vi "set initial operation mode.vi"(8 "error in (no error)":errorcluster, 11 "CCDCamera in":refnum<class "iKon-L.lvclass">) -> (0 "error out":errorcluster, 3 "CCDCamera out":refnum<class "iKon-L.lvclass">)   [LabVIEW 2018, in "iKon-L.lvclass"]
doc: "Write the current operation mode to the camera"
uses:
  iKon-L.lvclass
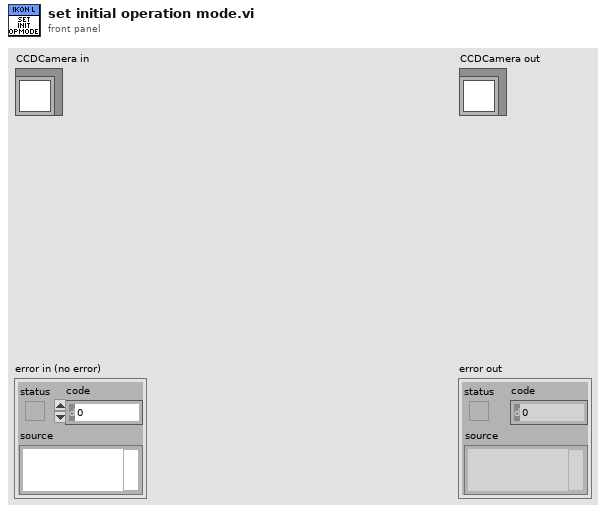
[diagram p1: front panel]
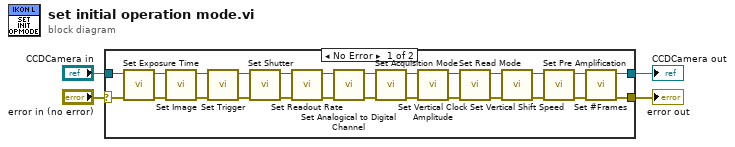
[diagram p0: block diagram]
diagram:
  n1 = case shown="No Error" "error in (no error)" {
    selector: "error in (no error)" -> [w14 w31]
    tunnel: "CCDCamera in" -> [w16 w32]
    tunnel: [w15 w32] -> w2
    tunnel: [w13 w31] -> w1
    frame No Error {
      n2 = call-dynamic "Set Exposure Time.vi"("error in (no error)"=w14, "CCDCamera in"=w16) -> ("error out"=w23:errorcluster, "CCDCamera out"=w30:refnum<class "iKon-L.lvclass">)  [unwired: 8 in]
      n3 = call-dynamic "Set Image.vi"("error in (no error)"=w23, "CCDCamera in"=w30) -> ("error out"=w22:errorcluster, "CCDCamera out"=w29:refnum<class "iKon-L.lvclass">)  [unwired: 8 in]
      n4 = call-dynamic "Set Trigger.vi"("error in (no error)"=w22, "CCDCamera in"=w29) -> ("error out"=w21:errorcluster, "CCDCamera out"=w28:refnum<class "iKon-L.lvclass">)  [unwired: 8 in]
      n5 = call-dynamic "Set Shutter.vi"("error in (no error)"=w21, "CCDCamera in"=w28) -> ("error out"=w8:errorcluster, "CCDCamera out"=w5:refnum<class "iKon-L.lvclass">)  [unwired: 8 in]
      n6 = call-dynamic "Set Readout Rate.vi"("error in (no error)"=w8, "CCDCamera in"=w5) -> ("error out"=w7:errorcluster, "CCDCamera out"=w6:refnum<class "iKon-L.lvclass">)  [unwired: 8 in]
      n7 = call-dynamic "Set Analogical to Digital Channel.vi"("error in (no error)"=w7, "CCDCamera in"=w6) -> ("error out"=w20:errorcluster, "CCDCamera out"=w27:refnum<class "iKon-L.lvclass">)  [unwired: 8 in]
      n8 = call-dynamic "Set Acquisition Mode.vi"("error in (no error)"=w20, "CCDCamera in"=w27) -> ("error out"=w19:errorcluster, "CCDCamera out"=w26:refnum<class "iKon-L.lvclass">)  [unwired: 8 in]
      n9 = call-dynamic "Set Vertical Clock Amplitude.vi"("error in (no error)"=w19, "CCDCamera in"=w26) -> ("error out"=w9:errorcluster, "CCDCamera out"=w10:refnum<class "iKon-L.lvclass">)  [unwired: 8 in]
      n10 = call-dynamic "Set Read Mode.vi"("error in (no error)"=w9, "CCDCamera in"=w10) -> ("error out"=w18:errorcluster, "CCDCamera out"=w25:refnum<class "iKon-L.lvclass">)  [unwired: 8 in]
      n11 = call-dynamic "Set Vertical Shift Speed.vi"("error in (no error)"=w18, "CCDCamera in"=w25) -> ("error out"=w11:errorcluster, "CCDCamera out"=w12:refnum<class "iKon-L.lvclass">)  [unwired: 8 in]
      n12 = call-dynamic "Set Pre Amplification.vi"("error in (no error)"=w11, "CCDCamera in"=w12) -> ("error out"=w17:errorcluster, "CCDCamera out"=w24:refnum<class "iKon-L.lvclass">)  [unwired: 8 in]
      n13 = call-dynamic "Set #Frames.vi"("error in (no error)"=w17, "CCDCamera in"=w24) -> ("error out"=w13:errorcluster, "CCDCamera out"=w15:refnum<class "iKon-L.lvclass">)  [unwired: 8 in]
    }
    frame Error {
    }
  }
  "error out" <- w1
  "CCDCamera out" <- w2
